vi "Logger Viewer.vi"(11 "error in (no error)":errorcluster) -> (15 "error out":errorcluster)   [LabVIEW 2018]
uses:
  Logger Global.vi
panel:
  out "Log Name":string
  out "Log File":string
  # "STATION LOG STATUS"
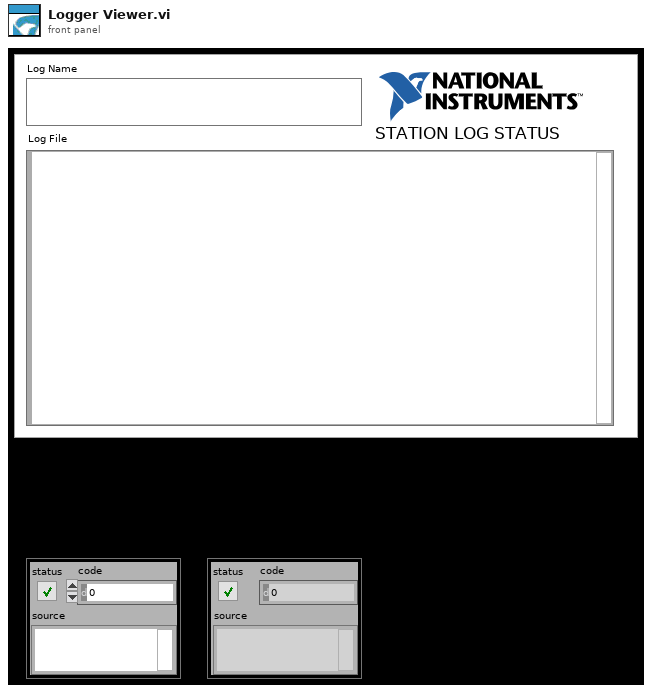
[diagram p1: front panel]
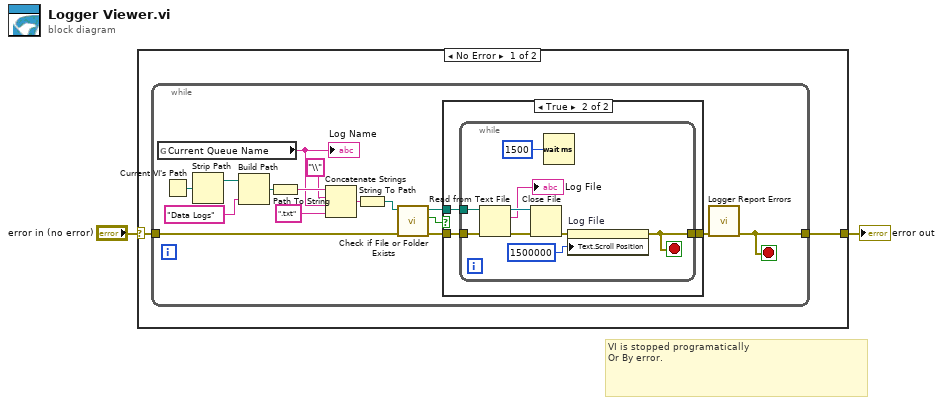
[diagram p0: block diagram]
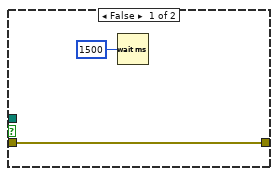
[diagram p2: hidden frame]
diagram:
  # "VI is stopped programatically\nOr By error."
  n1 = case shown="No Error" "error in (no error)" {
    selector: "error in (no error)" -> [w4 w35]
    tunnel: [w3 w35] -> w2
    frame No Error {
      n2 = while {
        tunnel: w4 -> [w9]
        tunnel: [w5] -> w3
        stop <- w5 stop-if-true
        n3 = global read "Logger Global.vi" "Current Queue Name"() -> (w13:string)
        "Log Name" <- w13
        n4 = Current VI's Path() -> (path=w17:path)
        n5 = Strip Path(path=w17) -> (stripped path=w20:path)  [unwired: 1 out]
        n6 = Build Path(base path=w20, name or relative path="Data Logs") -> (appended path=w19:path)
        n7 = Path To String(path=w19) -> (string=w15:string)
        n8 = Concatenate Strings(w15, "\\" ("string"), w13, ".txt" ("string")) -> (w12:string)
        n9 = String To Path(string=w12) -> (path=w7:path)
        n10 = call <vilib>:"Check if File or Folder Exists.vi"("error in (no error)"=w9, "path"=w7) -> ("error out"=w10:errorcluster, "file or folder exists?"=w6:bool, "dup path"=w8:path)  [unwired: 7 in]
        n11 = case shown="True" w6 {
          tunnel: [w21 w25] -> w11
          tunnel: w10 -> [w21 w24]
          tunnel: w8 -> [_ w23]
          frame False {
            n12 = Wait (ms)(milliseconds to wait=u32 1500) -> ()  [unwired: 1 out]
          }
          frame True {
            n13 = while {
              tunnel: w24 -> [w33]
              tunnel: [w26] -> w25
              tunnel: w23 -> [w30]
              stop <- w26 stop-if-true
              n14 = Read from Text File(file (use dialog)=w30, error in=w33) -> (refnum out=w31:refnum<file>, text=→"Log File":string, error out=w32:errorcluster)  [unwired: 2 in, 1 out]
              n15 = Close File(refnum=w31, error in=w32) -> (error out=w27:errorcluster)  [unwired: 1 out]
              n16 = Wait (ms)(milliseconds to wait=u32 1500) -> ()  [unwired: 1 out]
              n17 = property on="Log File" class="Str"(error in=w27, "Text.Scroll Position"=u32 1500000) -> (error out=w26:errorcluster)  [unwired: 1 in, 1 out]
            }
          }
        }
        n18 = call "Logger Report Errors.vi"("error in (no error)"=w11) -> ("error out"=w5:errorcluster)  [unwired: 14 in]
      }
    }
    frame Error {
    }
  }
  "error out" <- w2
